vi "washing machine server side.vi"() -> ()   [LabVIEW 2023]
panel:
  out "error out":errorcluster
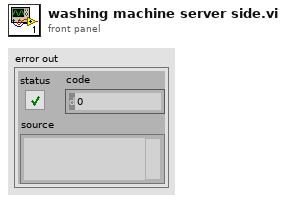
[diagram p1: front panel]
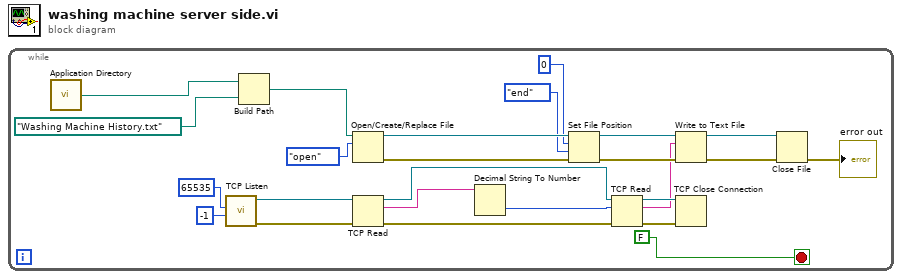
[diagram p0: block diagram]
diagram:
  n1 = while {
    stop <- FALSE stop-if-true
    n2 = call <vilib>:"Application Directory.vi"() -> ("Application Directory"=w14:path)
    n3 = call <vilib>:"TCP Listen.vi"("timeout ms (wait forever: -1)"=-1, "port"=u16 65535) -> ("error out"=w20:errorcluster, "connection ID"=w23:refnum<k5>)  [unwired: 5 in, 3 out]
    n4 = Build Path(base path=w14, name or relative path=path "Washing Machine History.txt") -> (appended path=w1:path)
    n5 = Open/Create/Replace File(file path (use dialog)=w1, operation (0:open)=enum16{"open"}."open") -> (refnum out=w10:refnum<file>, error out=w11:errorcluster)  [unwired: 4 in, 1 out]
    n6 = TCP Read(connection ID=w23, error in (no error)=w20) -> (connection ID out=w22:refnum<k5>, data out=w16:string, error out=w19:errorcluster)  [unwired: 3 in]
    n7 = Decimal String To Number(string=w16) -> (number=w15:i32)  [unwired: 2 in, 1 out]
    n8 = Set File Position(offset (in bytes) (0)=i64 0, refnum=w10, from (0:start)=enum16{"start", "end", "current"}."end", error in=w11) -> (refnum out=w7:refnum<file>, error out=w6:errorcluster)
    n9 = TCP Read(connection ID=w22, bytes to read=w15, error in (no error)=w19) -> (connection ID out=w21:refnum<k5>, data out=w5:string, error out=w18:errorcluster)  [unwired: 2 in]
    n10 = Write to Text File(file (use dialog)=w7, text=w5, error in=w6) -> (refnum out=w4:refnum<file>, error out=w3:errorcluster)  [unwired: 1 in, 1 out]
    n11 = TCP Close Connection(connection ID=w21, error in (no error)=w18) -> ()  [unwired: 1 in, 2 out]
    n12 = Close File(refnum=w4, error in=w3) -> (error out=→"error out":errorcluster)  [unwired: 1 out]
  }
